vi "sc_dir_build.vi"(8 "error in":errorcluster, 10 "Folder Name":string, 11 "Base Directory":path) -> (0 "error out":errorcluster, 3 "Created Folder":string)   [LabVIEW 2018]
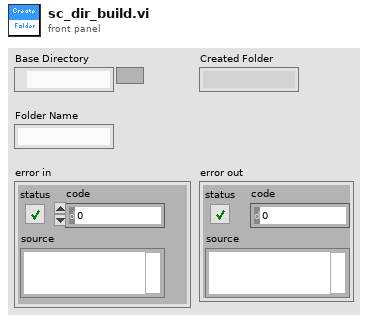
[diagram p1: front panel]
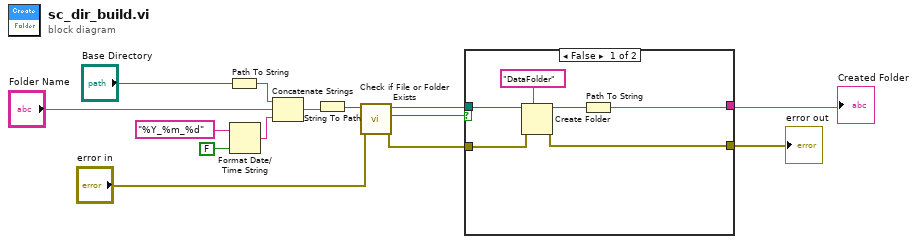
[diagram p0: block diagram]
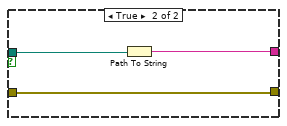
[diagram p2: hidden frame]
diagram:
  n1 = Path To String(path="Base Directory") -> (string=w5:string)
  n2 = Format Date/Time String(time format string (%c)="%Y_%m_%d", UTC format=FALSE) -> (date/time string=w6:string)  [unwired: 1 in]
  n3 = Concatenate Strings(w5, "Folder Name", w6) -> (w3:string)
  n4 = String To Path(string=w3) -> (path=w8:path)
  n5 = call <vilib>:"Check if File or Folder Exists.vi"("error in (no error)"="error in", "path"=w8) -> ("error out"=w11:errorcluster, "file or folder exists?"=w10:bool, "dup path"=w9:path)  [unwired: 7 in]
  n6 = case shown="False" w10 {
    tunnel: w9 -> [w18 w22]
    tunnel: w11 -> [w17 w23]
    tunnel: [w16 w23] -> w12
    tunnel: [w15 w21] -> w14
    frame False {
      n7 = Create Folder(prompt (Create Folder)="DataFolder", path (use dialog)=w18, error in=w17) -> (created path=w20:path, error out=w16:errorcluster)  [unwired: 1 out]
      n8 = Path To String(path=w20) -> (string=w15:string)
    }
    frame True {
      n9 = Path To String(path=w22) -> (string=w21:string)
    }
  }
  "Created Folder" <- w14
  "error out" <- w12
